vi "Position Tracking.vi"() -> ()   [LabVIEW 2017]
uses:
  Utility VIs/Refnum Names.vi
  <vilib>/Rock Robotics/WPI/ThirdParty/Phoenix-LabVIEW/Motor Controller/Get/CTRE_Phoenix_MotorController_GetSelectedSensorData.vi
  Globals/Position Data.vi
  <vilib>/Utility/file.llb/Read Delimited Spreadsheet (DBL).vi
  <vilib>/Rock Robotics/WPI/ThirdParty/Phoenix-LabVIEW/Pigeon IMU/CTRE_PigeonIMU_GetYPR.vi
panel:
  out "X and Y pos":cluster{dbl, dbl}(graph)
  out "Pigeon Yaw":cluster{"Yaw":dbl}(graph)
  out "XY Graph":cluster{"array":dbl[], "array":dbl[]}[](graph)
  out "Y position":dbl
  out "X position":dbl
  out "Dist from origin":dbl
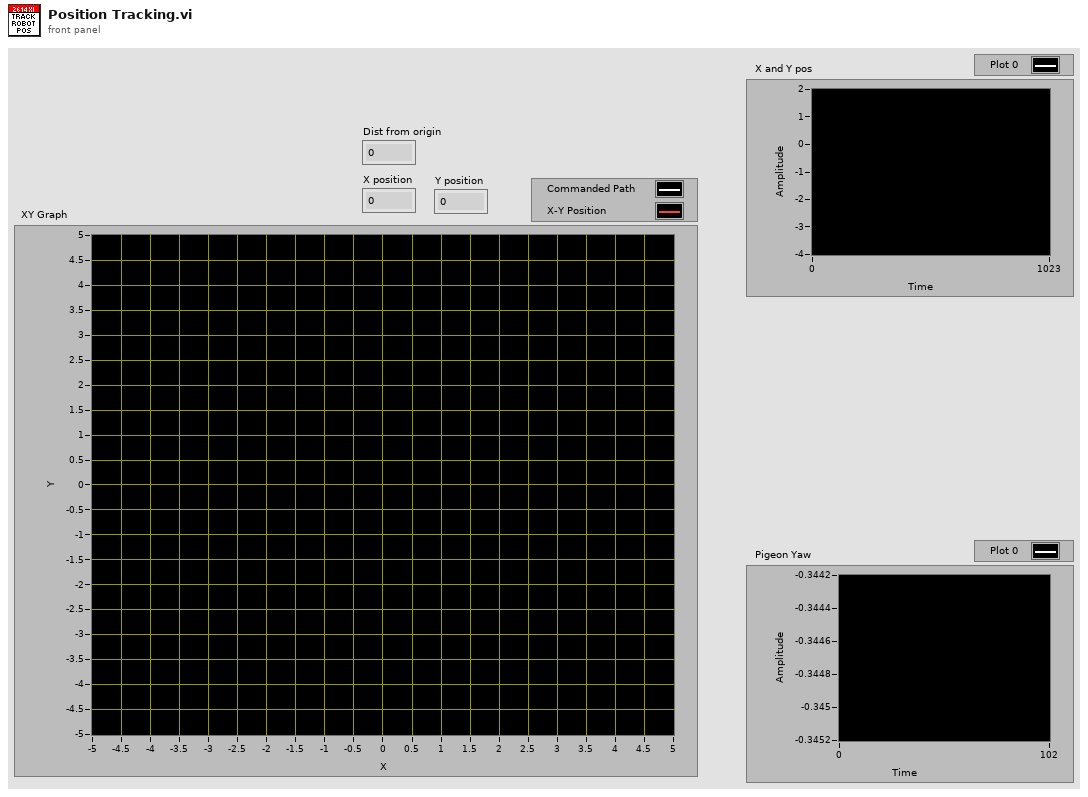
[diagram p1: front panel]
types:
  T1 = typedef "CTRE_PigeonIMU_DeviceRef.ctl" = cluster{"DeviceStatus":errorcluster, "Device Number":u8, "Type":T2, "Device ID":u32, "Handle":u64, "UsageFrame":u32, "Library Path":path}
  T2 = typedef "CTRE_PigeonIMU_ConnectionType.ctl" = u32
  T3 = typedef "WPI_MotorControlDeviceRef.ctl" = cluster{"DeviceStatus":errorcluster, "Type":T4, "PWM":cluster{"PWM Channel":T5, "DeadBand":T6}, "CAN":cluster{"Device Number":u8, "SetOutput VI Ref":variant, "GetOutput VI Ref":variant, "Enable VI Ref":variant, "Disable VI Ref":variant, "Data":variant}, "Invert":bool, "DIO PWM":cluster{"PWM \"Enable\" Channel":T5, "DIOChannel":T7, "PWM Rate":dbl}}
  T4 = typedef "WPI_MotorControlType.ctl" = enum16{"PWM", "CAN", "DIO PWM"}
  T5 = typedef "FPGA_DIOPWMChannel.ctl" = enum8{"PWM 0", "PWM 1", "PWM 2", "PWM 3", "PWM 4", "PWM 5", "PWM 6", "PWM 7", "PWM 8", "PWM 9", "PWM MXP 0", "PWM MXP 1", "PWM MXP 2", "PWM MXP 3", "PWM MXP 4", "PWM MXP 5", "PWM MXP 6", "PWM MXP 7", "PWM MXP 8", "PWM MXP 9", "Invalid"}
  T6 = typedef "WPI_PWMDeadband.ctl" = cluster{"Name":string, "maxPositivePwm":i32, "minPositivePwm":i32, "centerPwm":i32, "maxNegativePwm":i32, "minNegativePwm":i32, "angularRange":u16}
  T7 = typedef "FPGA_DIOChannel.ctl" = enum8{"DIO 0", "DIO 1", "DIO 2", "DIO 3", "DIO 4", "DIO 5", "DIO 6", "DIO 7", "DIO 8", "DIO 9", "DIO MXP 0", "DIO MXP 1", "DIO MXP 2", "DIO MXP 3", "DIO MXP 4", "DIO MXP 5", "DIO MXP 6", "DIO MXP 7", "DIO MXP 8", "DIO MXP 9", "DIO MXP 10", "DIO MXP 11", "DIO MXP 12", "DIO MXP 13", "DIO MXP 14", "DIO MXP 15", "SPI Port CS1", "SPI Port CS2", "SPI Port CS3", "SPI Port MISO", "SPI Port MOSI", "Invalid"}
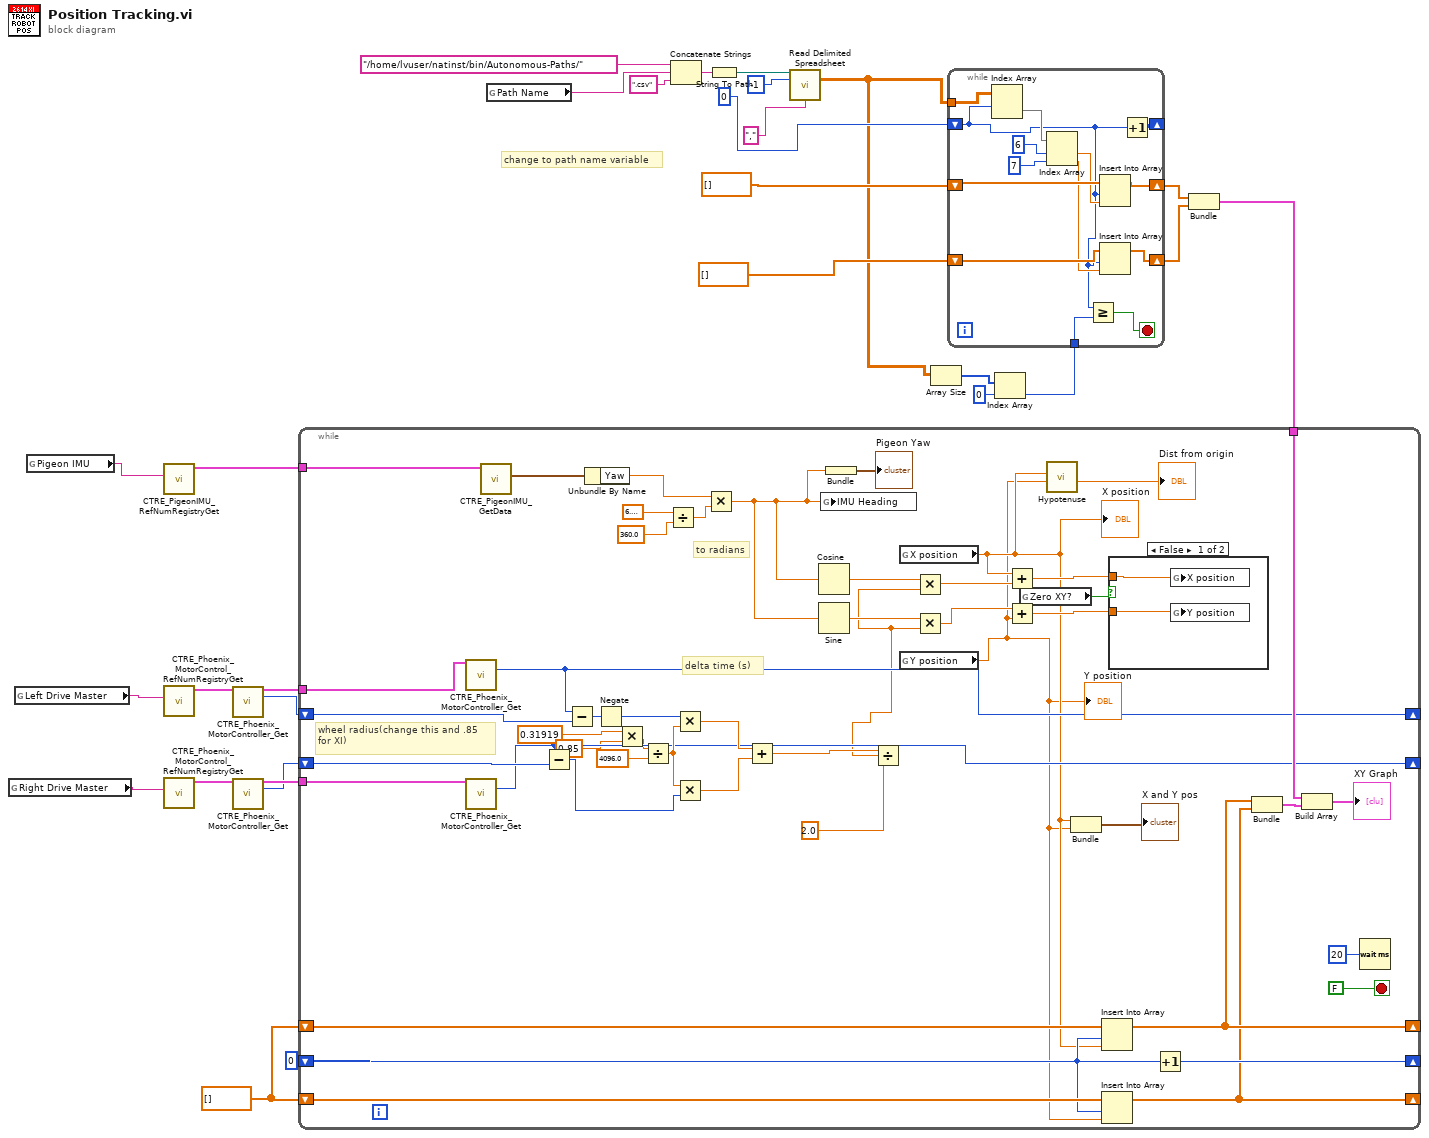
[diagram p0: block diagram]
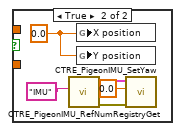
[diagram p2: hidden frame]
diagram:
  w27 = dbl[] [] ("array")
  # "change to path name variable"
  n1 = global read "Refnum Names.vi" "Right Drive Master"() -> (w4:string)
  n2 = global read "Refnum Names.vi" "Left Drive Master"() -> (w3:string)
  n3 = global read "Refnum Names.vi" "Pigeon IMU"() -> (w2:string)
  n4 = call <vilib>:"CTRE_PigeonIMU_RefNumRegistryGet.vi"("refnum name"=w2) -> ("PigeonIMUDevRef"=w29:T1)  [unwired: 9 in, 1 out]
  n5 = call <vilib>:"CTRE_Phoenix_MotorControl_RefNumRegistryGet.vi"("refnum name"=w3) -> ("PhoenixMotorControlDevRef"=w9:T3)  [unwired: 9 in, 1 out]
  n6 = call <vilib>:"CTRE_Phoenix_MotorControl_RefNumRegistryGet.vi"("refnum name"=w4) -> ("PhoenixMotorControlDevRef"=w8:T3)  [unwired: 9 in, 1 out]
  n7 = call-poly <vilib>:"CTRE_Phoenix_MotorController_Get.vi"("PhoenixMotorControlDevRef"=w9) -> ("PhoenixMotorControlDevRef"=w10:T3, "Position (Raw Sensor Units)"=w6:i32)  [unwired: 11 in, 2 out]
  n8 = call-poly <vilib>:"CTRE_Phoenix_MotorController_Get.vi"("PhoenixMotorControlDevRef"=w8) -> ("PhoenixMotorControlDevRef"=w7:T3, "Position (Raw Sensor Units)"=w5:i32)  [unwired: 11 in, 2 out]
  n9 = global read "Position Data.vi" "Path Name"() -> (w1:string)
  n10 = Concatenate Strings("/home/lvuser/natinst/bin/Autonomous-Paths/", w1, ".csv" ("string")) -> (w23:string)
  n11 = String To Path(string=w23) -> (path=w22:path)
  n12 = call-poly <vilib>:"Read Delimited Spreadsheet.vi"("file path (dialog if empty)"=w22, "number of rows (all:-1)"=-1, "delimiter (\\t)"="," ("delimiter (\\t)")) -> ("all rows"=w17:dbl[][])  [unwired: 7 in, 5 out]
  n13 = Array Size(array=w17) -> (size(s)=w16:i32[])
  n14 = Index Array(array=w16, index=0) -> (element=w14:i32)
  n15 = while {
    tunnel: w17 -> [w43]
    shift-right: [w42] -> _
    shift-left: 0 ("index (row)") -> [w33]
    shift-right: [w31] -> w13
    shift-left: dbl[] [] ("array") -> [w38]
    shift-right: [w30] -> w12
    shift-left: dbl[] [] ("array") -> [w37]
    tunnel: w14 -> [w34]
    stop <- w32 stop-if-true
    n16 = Index Array(array=w43, index (row)=w33) -> (element=w41:dbl[])  [unwired: 1 in]
    n17 = Index Array(array=w41, index #1=6 ("index"), index #2=7 ("index")) -> (element #1=w36:dbl, element #2=w35:dbl)
    n18 = Greater Or Equal?(x=w33, y=w34) -> (x >= y?=w32:bool)
    n19 = Insert Into Array(array=w38, index=w33, new element=w36) -> (w31:dbl[])
    n20 = Insert Into Array(array=w37, index=w33, new element=w35) -> (w30:dbl[])
    n21 = Increment(x=w33) -> (x+1=w42:i32)
  }
  n22 = Bundle("array"=w13, "array"=w12) -> (w11:cluster{"array":dbl[], "array":dbl[]})  [unwired: 1 in]
  n23 = while {
    tunnel: w29 -> [w90]
    shift-right: [w76] -> _
    shift-left: w27 -> [w80]
    shift-right: [w75] -> _
    shift-left: w27 -> [w79]
    shift-right: [w78] -> _
    shift-left: 0 ("index") -> [w77]
    tunnel: w11 -> [w72]
    tunnel: w10 -> [w71]
    tunnel: w7 -> [w70]
    shift-right: [w55] -> _
    shift-left: w6 -> [w56]
    shift-right: [w52] -> _
    shift-left: w5 -> [w54]
    stop <- FALSE stop-if-true
    # "wheel radius(change this and .85 for XI)"
    # "to radians"
    # "delta time (s)"
    n24 = call-poly <vilib>:"CTRE_Phoenix_MotorController_Get.vi"("PhoenixMotorControlDevRef"=w71) -> ("Position (Raw Sensor Units)"=w55:i32)  [unwired: 11 in, 3 out]
    n25 = call-poly <vilib>:"CTRE_Phoenix_MotorController_Get.vi"("PhoenixMotorControlDevRef"=w70) -> ("Position (Raw Sensor Units)"=w52:i32)  [unwired: 11 in, 3 out]
    n26 = call-poly <vilib>:"CTRE_PigeonIMU_GetData.vi"("PigeonIMUDevRef"=w90) -> ("Yaw Pitch Roll"=w89:cluster{"Yaw":dbl, "Pitch":dbl, "Roll":dbl})  [unwired: 8 in, 2 out]
    n27 = Subtract(x=w52, y=w54) -> (x-y=w57:i32)
    n28 = Subtract(x=w55, y=w56) -> (x-y=w63:i32)
    n29 = Unbundle By Name(w89) -> ("Yaw"=w66:dbl)
    n30 = Negate(x=w63) -> (-x=w53:i32)
    n31 = Multiply(x=0.31919, y=0.85) -> (x*y=w51:dbl)
    n32 = Divide(x=w51, y=4096.0) -> (x/y=w64:dbl)
    n33 = Divide(x=6.283185307179586, y=360.0) -> (x/y=w67:dbl)
    n34 = Multiply(x=w53, y=w64) -> (x*y=w59:dbl)
    n35 = Multiply(x=w64, y=w57) -> (x*y=w58:dbl)
    n36 = Multiply(x=w66, y=w67) -> (x*y=w48:dbl)
    n37 = Add(x=w59, y=w58) -> (x+y=w61:dbl)
    n38 = Cosine(x=w48) -> (cos(x)=w88:dbl)
    n39 = Sine(x=w48) -> (sin(x)=w86:dbl)
    n40 = global write "Position Data.vi" "IMU Heading"(w48) -> ()
    n41 = Bundle(w48) -> (→"Pigeon Yaw":cluster{dbl})  [unwired: 1 in]
    n42 = Divide(x=w61, y=2.0) -> (x/y=w44:dbl)
    n43 = global read "Position Data.vi" "X position"() -> (w47:dbl)
    "X position" <- w47
    n44 = global read "Position Data.vi" "Y position"() -> (w46:dbl)
    "Y position" <- w46
    n45 = Multiply(x=w88, y=w44) -> (x*y=w87:dbl)
    n46 = Multiply(x=w86, y=w44) -> (x*y=w85:dbl)
    n47 = Add(x=w47, y=w87) -> (x+y=w83:dbl)
    n48 = Add(x=w85, y=w46) -> (x+y=w82:dbl)
    n49 = global read "Position Data.vi" "Zero XY?"() -> (w49:bool)
    n50 = call "Hypotenuse.vi"("b"=w46, "a"=w47) -> ("c"=→"Dist from origin":dbl)  [unwired: 9 in]
    n51 = Bundle("X position"=w47, "Y position"=w46) -> (→"X and Y pos":cluster{"X position":dbl, "Y position":dbl})  [unwired: 1 in]
    n52 = Insert Into Array(array=w80, index=w77, new element=w47) -> (w76:dbl[])
    n53 = Insert Into Array(array=w79, index=w77, new element=w46) -> (w75:dbl[])
    n54 = case shown="False" w49 {
      tunnel: w83 -> [w94 _]
      tunnel: w82 -> [w93 _]
      frame False {
        n55 = global write "Position Data.vi" "X position"(w94) -> ()
        n56 = global write "Position Data.vi" "Y position"(w93) -> ()
      }
      frame True {
        w99 = 0.0 ("X position")
        n57 = call <vilib>:"CTRE_PigeonIMU_RefNumRegistryGet.vi"("refnum name"="IMU") -> ("error out"=w96:errorcluster, "PigeonIMUDevRef"=w95:T1)  [unwired: 9 in]
        n58 = global write "Position Data.vi" "X position"(w99) -> ()
        n59 = global write "Position Data.vi" "Y position"(w99) -> ()
        n60 = call <vilib>:"CTRE_PigeonIMU_SetYaw.vi"("error in (no error)"=w96, "Value"=0.0, "PigeonIMUDevRef"=w95) -> ()  [unwired: 7 in, 2 out]
      }
    }
    n61 = Increment(x=w77) -> (x+1=w78:i32)
    n62 = Bundle("array"=w76, "array"=w75) -> (w74:cluster{"array":dbl[], "array":dbl[]})  [unwired: 1 in]
    n63 = Build Array(w72, w74) -> (→"XY Graph":cluster{"array":dbl[], "array":dbl[]}[])
    n64 = Wait (ms)(milliseconds to wait=u32 20) -> ()  [unwired: 1 out]
  }
